vi "Realtime XY Graph.vi"() -> ()   [LabVIEW 2014]
panel:
  in  "stop":bool
  out "XY Graph":cluster{"Y":dbl[], "Y":dbl[]}[](graph)
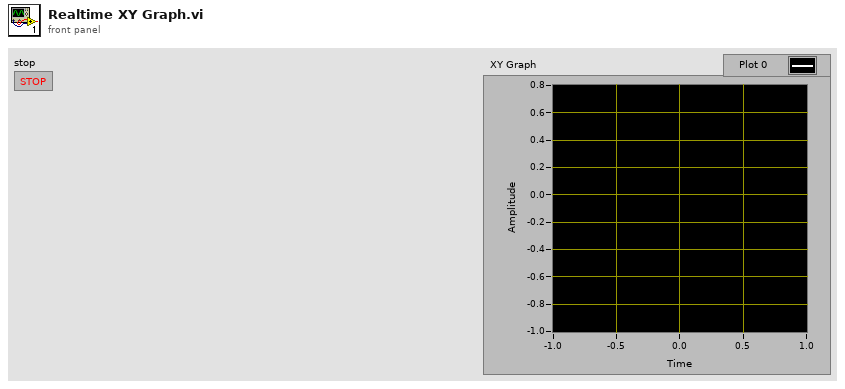
[diagram p1: front panel]
types:
  T1 = cluster{"Roll":dbl, "Pitch":dbl, "Vertical Speed":dbl, "Yaw Speed":dbl}
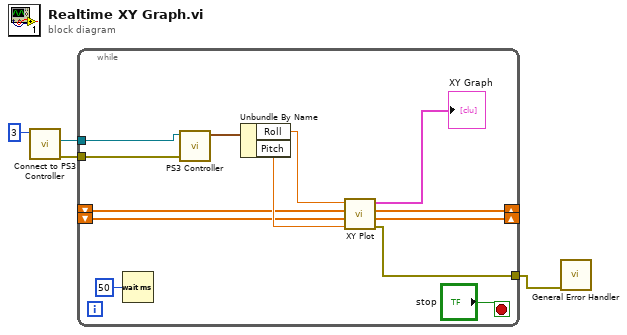
[diagram p0: block diagram]
diagram:
  n1 = call "Connect to PS3 Controller.vi"("device ID"=3) -> ("error out"=w4:errorcluster, "device ID 2"=w3:refnum<k1>)  [unwired: 7 in, 1 out]
  n2 = while {
    tunnel: w4 -> [w17]
    tunnel: w3 -> [w16]
    tunnel: [w11] -> w1
    shift-right: [w9] -> _
    shift-left: _ -> [w7]
    shift-right: [w8] -> _
    shift-left: _ -> [w6]
    stop <- "stop" stop-if-true
    n3 = Wait (ms)(milliseconds to wait=u32 50) -> ()  [unwired: 1 out]
    n4 = call "PS3 Controller.vi"("error in (no error)"=w17, "device ID"=w16) -> ("Control cluster"=w15:T1)  [unwired: 6 in, 3 out]
    n5 = Unbundle By Name(w15) -> ("Roll"=w14:dbl, "Pitch"=w13:dbl)
    n6 = call "XY Plot.vi"("X"=w14, "X array"=w7, "Y array"=w6, "Y"=w13) -> ("XY Graph"=→"XY Graph":cluster{"Y":dbl[], "Y":dbl[]}[], "X array"=w9:dbl[], "Y array"=w8:dbl[], "error out"=w11:errorcluster)  [unwired: 2 in]
  }
  n7 = call <vilib>:"General Error Handler.vi"("error in (no error)"=w1) -> ()  [unwired: 10 in, 5 out]
